vi "CoriEngine.vi"(0 "object in":refnum<class "CoriFlowBFS1Plus.lvclass">, 2 "Sample Rate (Hz)":dbl=10.0 format="%#_13g", 5 "error in (no error)":errorcluster) -> (14 "object out":refnum<class "CoriFlowBFS1Plus.lvclass">, 19 "error out":errorcluster)   [LabVIEW 2021, in "CoriFlowBFS1Plus.lvclass"]
uses:
  CoriFlowBFS1Plus.lvclass
  CoriFlowBFS1Plus.lvclass/CoriFlowBFS1Plus.ctl
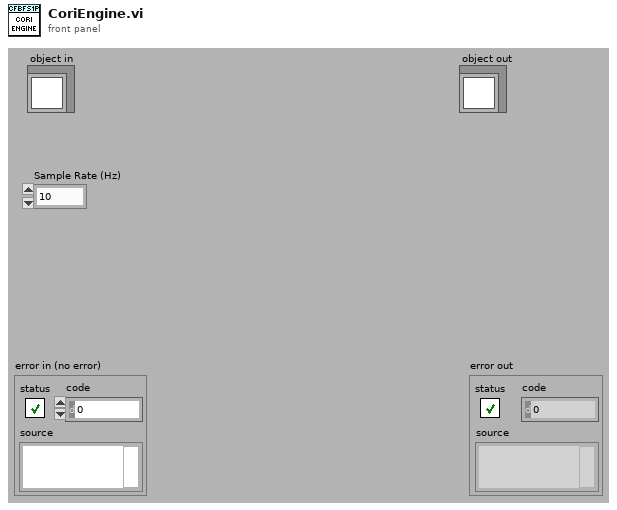
[diagram p1: front panel]
types:
  T1 = cluster{"Message":string, "Message Data":variant}
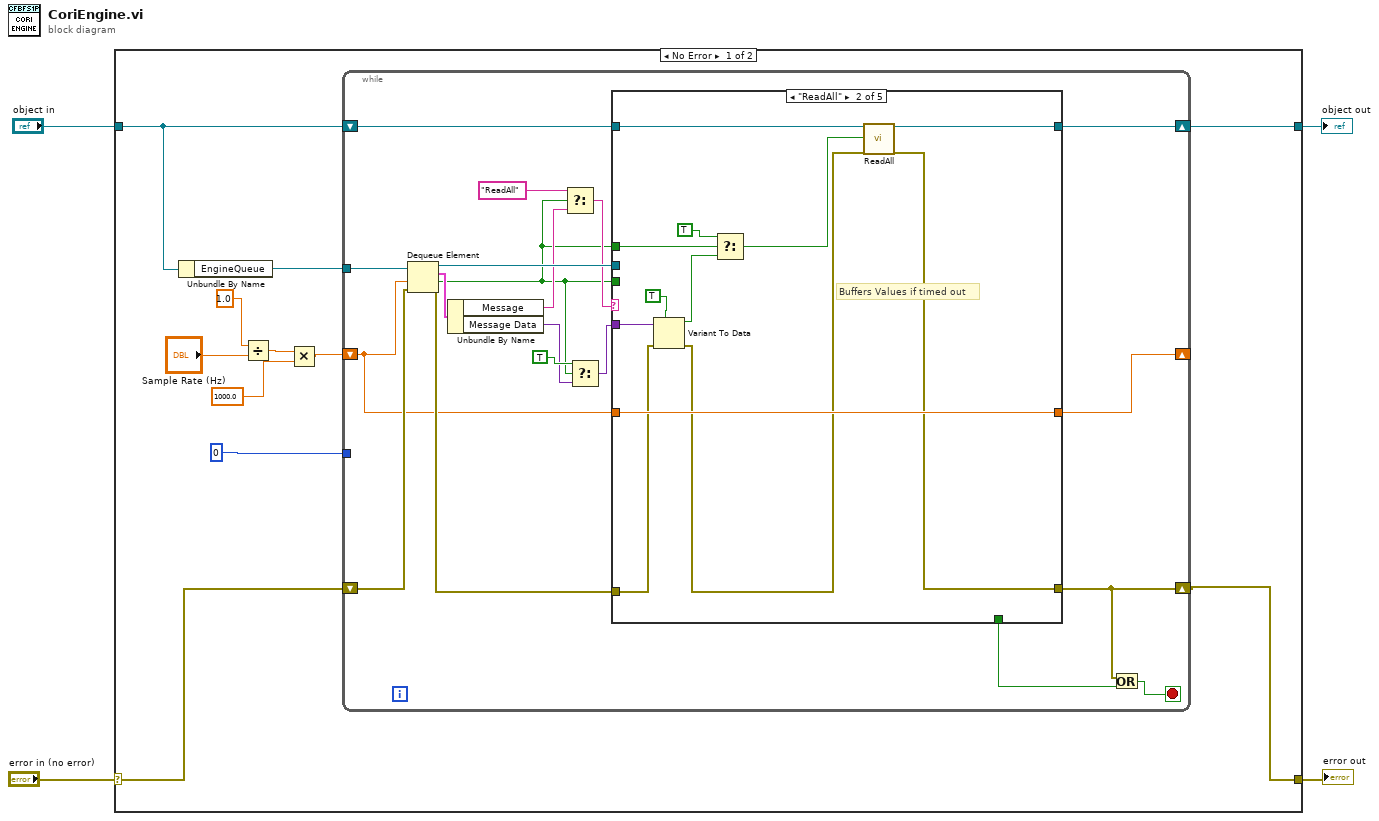
[diagram p0: block diagram]
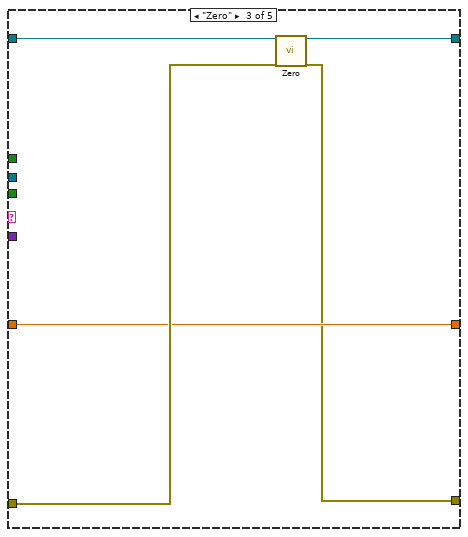
[diagram p3: hidden frame]
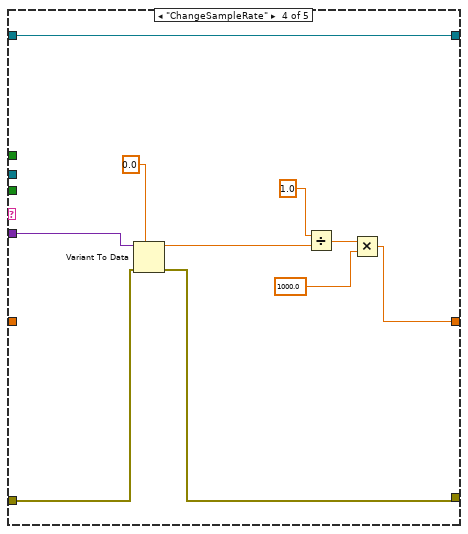
[diagram p4: hidden frame]
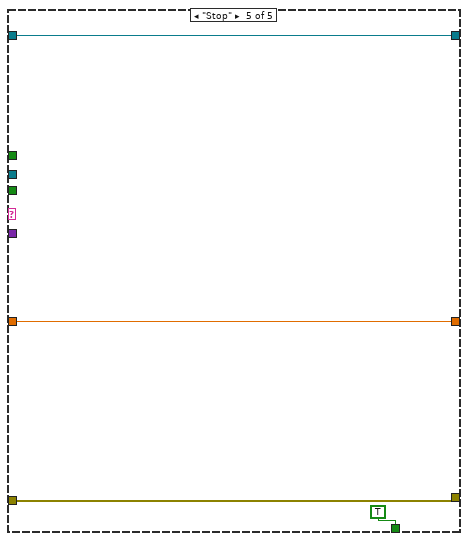
[diagram p5: hidden frame]
diagram:
  n1 = case shown="No Error" "error in (no error)" {
    selector: "error in (no error)" -> [w7 w70]
    tunnel: [w6 w70] -> w3
    tunnel: [w14 w69] -> w1
    tunnel: "object in" -> [w15 w69]
    frame No Error {
      n2 = Unbundle By Name(w15) -> ("EngineQueue"=w5:refnum<queue>)
      n3 = Divide(x=1.0, y="Sample Rate (Hz)") -> (x/y=w10:dbl)
      n4 = Multiply(x=w10, y=1000.0) -> (x*y=w8:dbl)
      n5 = while {
        shift-right: [w26] -> w14
        shift-left: w15 -> [w27]
        tunnel: w5 -> [w34]
        shift-right: [w29] -> w6
        shift-left: w7 -> [w32]
        tunnel: u32 0 ("millisecond multiple") -> [_]
        shift-right: [w25] -> _
        shift-left: w8 -> [w23]
        stop <- w30 stop-if-true
        n6 = Dequeue Element(queue=w34, timeout in ms (-1)=w23, error in (no error)=w32) -> (queue out=w24:refnum<queue>, element=w33:T1, timed out?=w18:bool, error out=w31:errorcluster)
        n7 = Unbundle By Name(w33) -> ("Message"=w20:string, "Message Data"=w17:variant)
        n8 = Select(t="ReadAll", s=w18, f=w20) -> (s? t:f=w22:string)
        n9 = Select(t=TRUE, s=w18, f=w17) -> (s? t:f=w16:variant)
        n10 = case shown="\"ReadAll\"" w22 {
          tunnel: w24 -> [_ _ _ _ _]
          tunnel: w31 -> [w37 w43 w54 w61 w68]
          tunnel: [w37 w46 w50 w62 w68] -> w29
          tunnel: [_ _ _ _ TRUE] -> w28
          tunnel: [w36 w49 w51 w64 w66] -> w26
          tunnel: w27 -> [w36 w48 w52 w64 w66]
          tunnel: w23 -> [w35 w47 w53 _ w65]
          tunnel: [w35 w47 w53 w56 w65] -> w25
          tunnel: w16 -> [_ w45 _ w55 _]
          tunnel: w18 -> [_ _ _ _ _]
          tunnel: w18 -> [_ w41 _ _ _]
          frame "False", Default {
          }
          frame "ReadAll" {
            # "Buffers Values if timed out"
            n11 = Variant To Data(error in=w43, type=TRUE, Variant=w45) -> (data=w38:bool, error out=w44:errorcluster)
            n12 = Select(t=TRUE, s=w41, f=w38) -> (s? t:f=w39:bool)
            n13 = call-dynamic "ReadAll.vi"("object in"=w48, "Buffer Values?"=w39, "error in (no error)"=w44) -> ("object out"=w49:refnum<class "CoriFlowBFS1Plus.lvclass">, "error out"=w46:errorcluster)  [unwired: 14 in, 1 out]
          }
          frame "Zero" {
            n14 = call-dynamic "Zero.vi"("object in"=w52, "error in (no error)"=w54) -> ("object out"=w51:refnum<class "CoriFlowBFS1Plus.lvclass">, "error out"=w50:errorcluster)  [unwired: 16 in]
          }
          frame "ChangeSampleRate" {
            n15 = Variant To Data(error in=w61, type=0.0, Variant=w55) -> (data=w57:dbl, error out=w62:errorcluster)
            n16 = Divide(x=1.0, y=w57) -> (x/y=w59:dbl)
            n17 = Multiply(x=w59, y=1000.0) -> (x*y=w56:dbl)
          }
          frame "Stop" {
          }
        }
        n18 = Or(x=w29, y=w28) -> (x .or. y?=w30:bool)
      }
    }
    frame Error {
    }
  }
  "error out" <- w3
  "object out" <- w1
